vi "Table Highlight.vi"(7 "Action":enum16{"Reset", "Highlight 1 Row"}(ring), 8 "error in":errorcluster, 9 "Color Box":u32(colorbox)=16776960, 10 "Row":i32, 11 "Table Ref in":refnum<vi>) -> (0 "error out":errorcluster, 3 "Table Ref out":refnum<vi>)   [LabVIEW 2023, in "FPT Framework UI.lvlib"]
doc: "Use this VI to reset the highlight or to highlight a specific row."
uses:
  FPT Framework UI.lvlib
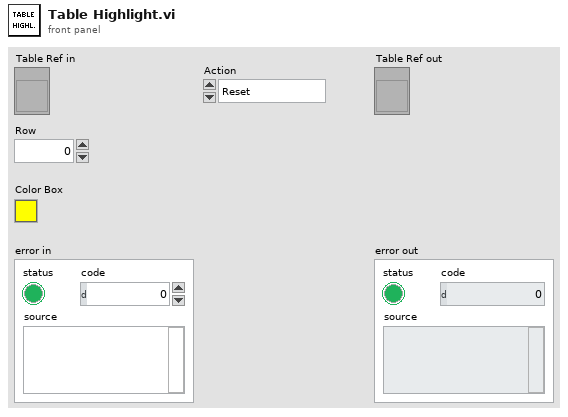
[diagram p1: front panel]
types:
  T1 = typedef "LVRowAndColumnTypeDef.ctl" = cluster{"Row":i32, "Column":i32}
  T2 = typedef "LVRowAndColumnUnsignedTypeDef.ctl" = cluster{"Row":u32, "Column":u32}
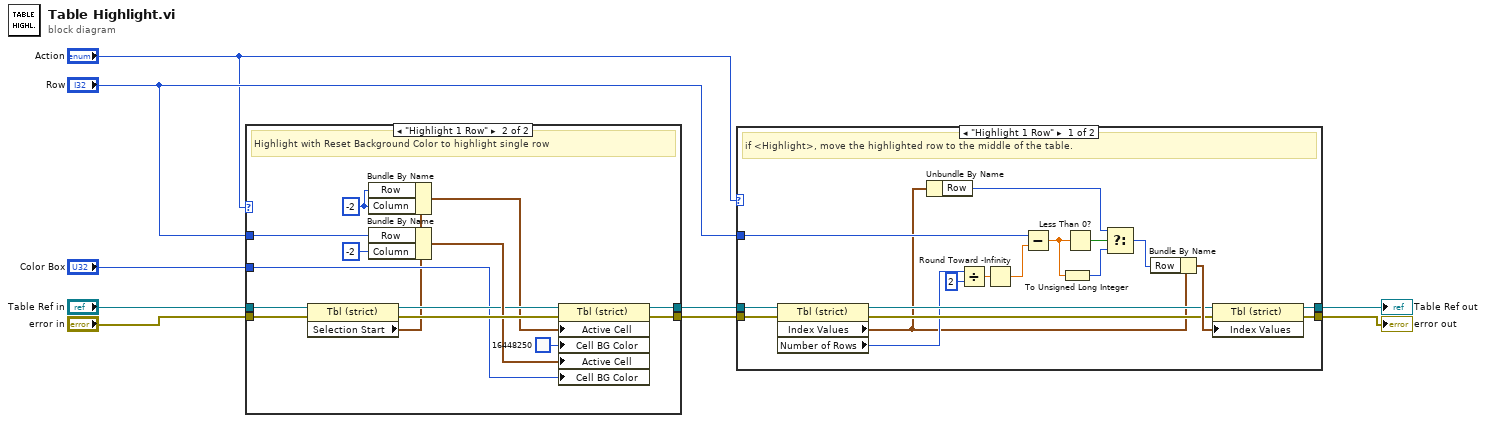
[diagram p0: block diagram]
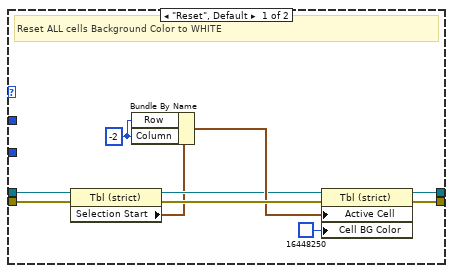
[diagram p2: hidden frame]
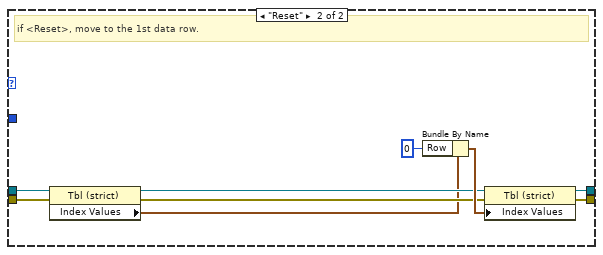
[diagram p3: hidden frame]
diagram:
  n1 = case shown="\"Highlight 1 Row\"" "Action" {
    tunnel: "error in" -> [w19 w33]
    tunnel: "Table Ref in" -> [w15 w29]
    tunnel: "Color Box" -> [_ w28]
    tunnel: [w14 w27] -> w6
    tunnel: [w13 w26] -> w5
    tunnel: "Row" -> [_ w25]
    frame "Reset", Default {
      w11 = -2 ("Column")
      # "Reset ALL cells Background Color to WHITE"
      n2 = property on="Property Node" class="Tbl (strict)"(reference=w15, error in=w19) -> (reference out=w16:refnum<vi>, error out=w18:errorcluster, "Selection Start"=w12:T1)
      n3 = Bundle By Name(cluster=w12, "Row"=w11, "Column"=w11) -> (w17:T1)
      n4 = property on="Property Node" class="Tbl (strict)"(reference=w16, error in=w18, "Active Cell"=w17, "Cell BG Color"=u32 16448250 ("Active Cell:Cell Background Color")) -> (reference out=w14:refnum<vi>, error out=w13:errorcluster)
    }
    frame "Highlight 1 Row" {
      w21 = -2 ("Column")
      # "Highlight with Reset Background Color to highlight single row"
      n5 = property on="Property Node" class="Tbl (strict)"(reference=w29, error in=w33) -> (reference out=w30:refnum<vi>, error out=w32:errorcluster, "Selection Start"=w23:T1)
      n6 = Bundle By Name(cluster=w23, "Row"=w21, "Column"=w21) -> (w22:T1)
      n7 = Bundle By Name(cluster=w23, "Row"=w25, "Column"=-2) -> (w31:T1)
      n8 = property on="Property Node" class="Tbl (strict)"(reference=w30, error in=w32, "Active Cell"=w22, "Cell BG Color"=u32 16448250 ("Active Cell:Cell Background Color"), "Active Cell"=w31, "Cell BG Color"=w28) -> (reference out=w27:refnum<vi>, error out=w26:errorcluster)
    }
  }
  n9 = case shown="\"Highlight 1 Row\"" "Action" {
    tunnel: w6 -> [w51 w60]
    tunnel: w5 -> [w50 w59]
    tunnel: [w46 w55] -> w4
    tunnel: [w45 w54] -> w3
    tunnel: "Row" -> [w44 _]
    frame "Highlight 1 Row" {
      # "if <Highlight>, move the highlighted row to the middle of the table."
      n10 = property on="Property Node" class="Tbl (strict)"(reference=w51, error in=w50) -> (reference out=w48:refnum<vi>, error out=w47:errorcluster, "Index Values"=w41:T2, "Number of Rows"=w43:u32)
      n11 = Unbundle By Name(w41) -> ("Row"=w34:u32)
      n12 = Divide(x=w43, y=u32 2) -> (x/y=w39:dbl)
      n13 = Round Toward -Infinity(1:w39) -> (0:w38:dbl)
      n14 = Subtract(x=w44, y=w38) -> (x-y=w36:dbl)
      n15 = To Unsigned Long Integer(number=w36) -> (unsigned 32bit integer=w35:u32)
      n16 = Less Than 0?(x=w36) -> (x < 0?=w37:bool)
      n17 = Select(t=w34, s=w37, f=w35) -> (s? t:f=w42:u32)
      n18 = Bundle By Name(cluster=w41, "Row"=w42) -> (w49:T2)
      n19 = property on="Property Node" class="Tbl (strict)"(reference=w48, error in=w47, "Index Values"=w49) -> (reference out=w46:refnum<vi>, error out=w45:errorcluster)
    }
    frame "Reset" {
      # "if <Reset>, move to the 1st data row."
      n20 = property on="Property Node" class="Tbl (strict)"(reference=w60, error in=w59) -> (reference out=w57:refnum<vi>, error out=w56:errorcluster, "Index Values"=w53:T2)
      n21 = Bundle By Name(cluster=w53, "Row"=u32 0) -> (w58:T2)
      n22 = property on="Property Node" class="Tbl (strict)"(reference=w57, error in=w56, "Index Values"=w58) -> (reference out=w55:refnum<vi>, error out=w54:errorcluster)
    }
  }
  "error out" <- w3
  "Table Ref out" <- w4
